vi "Select REG to RB.vi"(6 "length":i32=1, 7 "offset":i32=3, 8 "Error In":errorcluster, 11 "Manual Write":string) -> (0 "Error Out":errorcluster, 3 "Readback":string)   [LabVIEW 2017]
uses:
  <vilib>/Utility/error.llb/whitespace.ctl
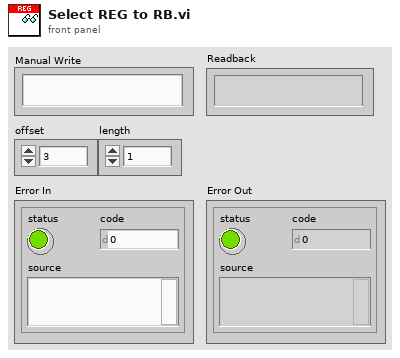
[diagram p1: front panel]
types:
  T1 = typedef "whitespace.ctl" = u16
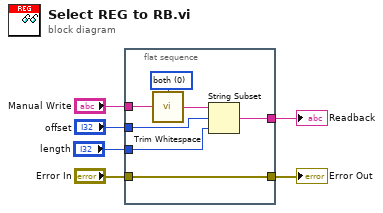
[diagram p0: block diagram]
diagram:
  n1 = flat-sequence {
    tunnel: "Manual Write" -> [w13]
    tunnel: [w8] -> w1
    tunnel: "Error In" -> [w11]
    tunnel: [w11] -> w4
    tunnel: "offset" -> [w10]
    tunnel: "length" -> [w9]
    frame #0 {
      w12 = T1 0 items=["both", "start of string", "end of string"] ("location (both)")
      n2 = call <vilib>:"Trim Whitespace.vi"("string"=w13, "location (both)"=w12) -> ("trimmed string"=w7:string)
      n3 = String Subset(string=w7, offset (0)=w10, length (rest)=w9) -> (substring=w8:string)
    }
  }
  "Readback" <- w1
  "Error Out" <- w4
